vi "Sig2MS SigProc.vi"(8 "error in (no error)":errorcluster, 9 "Signal in":waveform(sgl), 11 "Sig2MS in":refnum<class "Sig2MS.lvclass">) -> (0 "error out":errorcluster, 1 "Signal out":waveform(sgl), 3 "Sig2MS out":refnum<class "Sig2MS.lvclass">)   [LabVIEW 2018, in "Sig2MS.lvclass"]
uses:
  Sig2MS.lvclass
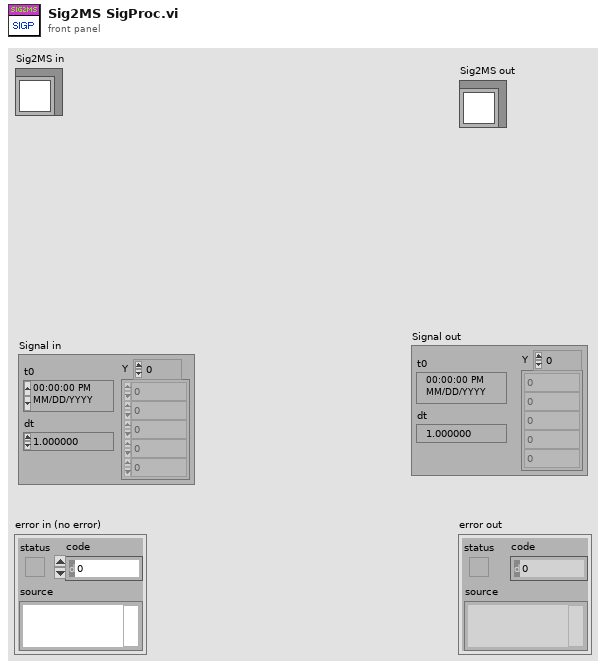
[diagram p1: front panel]
types:
  T1 = cluster{"startTime":dbl, "scanData":cluster{"dt":dbl, "xdata":dbl[], "ydata":sgl[], "beta":dbl[]}[], "xyXLabel":string, "xyYLabel":string, "wfmXLabel":string, "wfmYLabel":string, "ionData":cluster{"dt":dbl, "ydata":sgl[]}[], "ionXLabel":string, "ionYLabel":string}
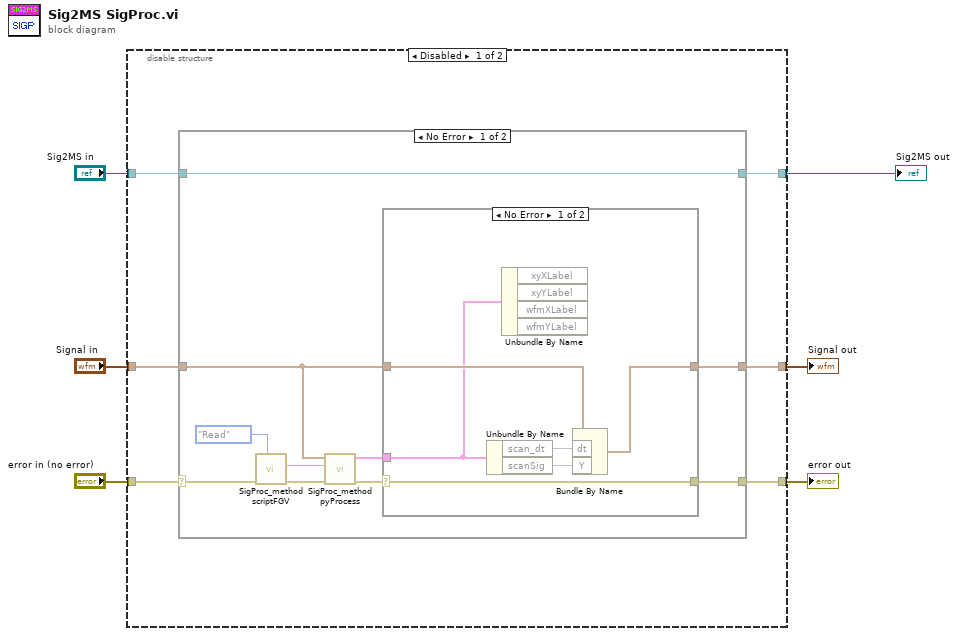
[diagram p0: block diagram]
diagram:
  n1 = disable-structure shown="Disabled" {
    disable-tunnel: "error in (no error)" -> [w12 _]
    disable-tunnel: "Sig2MS in" -> [w11 _]
    disable-tunnel: "Signal in" -> [w10 _]
    disable-tunnel: [w9 _] -> w3
    disable-tunnel: [w8 _] -> w2
    disable-tunnel: [w7 _] -> w1
    frame Disabled {
      n2 = case shown="No Error" w12 {
        selector: w12 -> [w18 w37]
        tunnel: [w15 w37] -> w9
        tunnel: [w22 w36] -> w7
        tunnel: w11 -> [w22 w36]
        tunnel: w10 -> [w13 w35]
        tunnel: [w20 w35] -> w8
        frame No Error {
          n3 = call "SigProc_method scriptFGV.vi"("Function"=enum16{"Read", "Write", "Init"}."Read", "error in"=w18) -> ("error out"=w19:errorcluster, "Script out"=w14:string)  [unwired: 6 in]
          n4 = call "SigProc_method pyProcess.vi"("error in (no error)"=w19, "newScriptCode"=w14, "dataParam"=w13) -> ("error out"=w16:errorcluster, "newSigInfo"=w17:T1)  [unwired: 5 in, 2 out]
          n5 = case shown="No Error" w16 {
            selector: w16 -> [w32 w34]
            tunnel: w13 -> [w31 w33]
            tunnel: [w28 w33] -> w20
            tunnel: w17 -> [w27 _]
            tunnel: [w32 w34] -> w15
            frame No Error {
              n6 = Unbundle By Name(w27) -> ("scan_dt"=w29, "scanSig"=w30)
              n7 = Unbundle By Name(w27) -> ("xyXLabel"=w26:string, "xyYLabel"=w25:string, "wfmXLabel"=w24:string, "wfmYLabel"=w23:string)
              n8 = Bundle By Name(cluster=w31, "dt"=w29, "Y"=w30) -> (w28:waveform(sgl))
            }
            frame Error {
            }
          }
        }
        frame Error {
        }
      }
    }
    frame Enabled {
    }
  }
  "error out" <- w3
  "Sig2MS out" <- w1
  "Signal out" <- w2
